vi "PH_SHS_Analysis_Statistician.panel.vi"(0 "object ref":refnum<vi>, 5 "error in (no error)":errorcluster) -> (19 "error out":errorcluster)   [LabVIEW 2014, in "PH_SHS_Analysis_Statistician.lvlib"]
doc: "This is just an example for a GUI thread.\n\nLicense Agreement for this software:\n\nCopyright (C)\nGesellschaft für Schwerionenforschung, GSI\nPlanckstr. 1\n64291 Darmstadt\nGermany\n\nContact: D.Beck@gsi.de \n\nThis program is free software; you can redistribute it and/or modify it under the terms of the GNU General Public License as published by the Free Software Foundation; either version 2 of the license, or (at your option) any later version.\n\nThis program is distributed in the hope that it will be useful, but WITHOUT ANYW ARRANTY; without even the implied warranty of MERCHANTABILITY or FITNESS FOR A PARTICULAR PURPOSE. See the GNU General License for more details (http://www.gnu.org).\n\nGesellschaft für Schwerionenforschung, GSI\nPlanckstr. 1, 64291 Darmstadt, Germany\nFor all questions and ideas contact: M.Richter@gsi.de, H.Brand@gsi.de or D.Beck@gsi.de.\nLast update: 18-DEC-2002"
uses:
  PH_SHS_Analysis_Statistician.lvlib
  PH_SHS_Analysis/PH_SHS_Analysis.Zernike Coefficients.ctl
  PH_Basics/PH_Common/PH_Common.lvlib
  CS_Core/CSSystem/CSSystemLib/CSSystemLib.lvlib
  PH_SHS_Analysis/PH_SHS_Analysis.lvlib
  PH_Basics/PH_Class/PH_Class.lvlib
panel:
  in  "Sample Length":i32=1
  in  "Clear Data":bool
  out "Current PtV [Lambda]":dbl
  out "Current Zernike Coefficients":T1 {"2nd Spherical" scale=-2.0..2.0 scale format="%.2f"; "2nd Coma y" scale=-2.0..2.0 scale format="%.2f"; "2nd Coma x" scale=-2.0..2.0 scale format="%.2f"; "2nd Astig 45°" scale=-2.0..2.0 scale format="%.2f"; "2nd Astig 0°" scale=-2.0..2.0 scale format="%.2f"; "Trefoil 30°" scale=-2.0..2.0 scale format="%.2f"; "Trefoil 0°" scale=-2.0..2.0 scale format="%.2f"; "Spherical" scale=-2.0..2.0 scale format="%.2f"; "Coma y" scale=-2.0..2.0 scale format="%.2f"; "Coma x" scale=-2.0..2.0 scale format="%.2f"; "Astig 45°" scale=-2.0..2.0 scale format="%.2f"; "Astig 0°" scale=-2.0..2.0 scale format="%.2f"; "Defocus" scale=-2.0..2.0 scale format="%.2f"; "Tilt y" scale=-2.0..2.0 scale format="%.2f"; "Tilt x" scale=-2.0..2.0 scale format="%.2f"}
  in  "Stat or Trend":bool
  in  "Export Data":bool
  out "Result Graph":cluster{dbl[], dbl[]}[](graph)
  out "Std Dev Data 3":dbl caption="Unit" format="%#_4g"
  in  "Dummy Std Dev":string caption="Std Dev"
  in  "Dummy Mean":string caption="Mean"
  out "Mean Data 3":dbl caption="Unit" format="%#_4g"
  out "Std Dev Data 2":dbl caption="Unit" format="%#_4g"
  out "Mean Data 2":dbl caption="Unit" format="%#_4g"
  out "Std Dev Data 1":dbl caption="Unit" format="%#_4g"
  out "Mean Data 1":dbl caption="Unit" format="%#_4g"
  in  "Data 3":u16(ring) items=["nothing "]
  in  "Data 2":u16(ring) items=["nothing "]
  in  "Data 1":u16(ring) items=["nothing "]
  out "Status":u32(colorbox)
  in  "Operator":string
  in  "Delete":bool
  # "PCS"
  # "3.40"
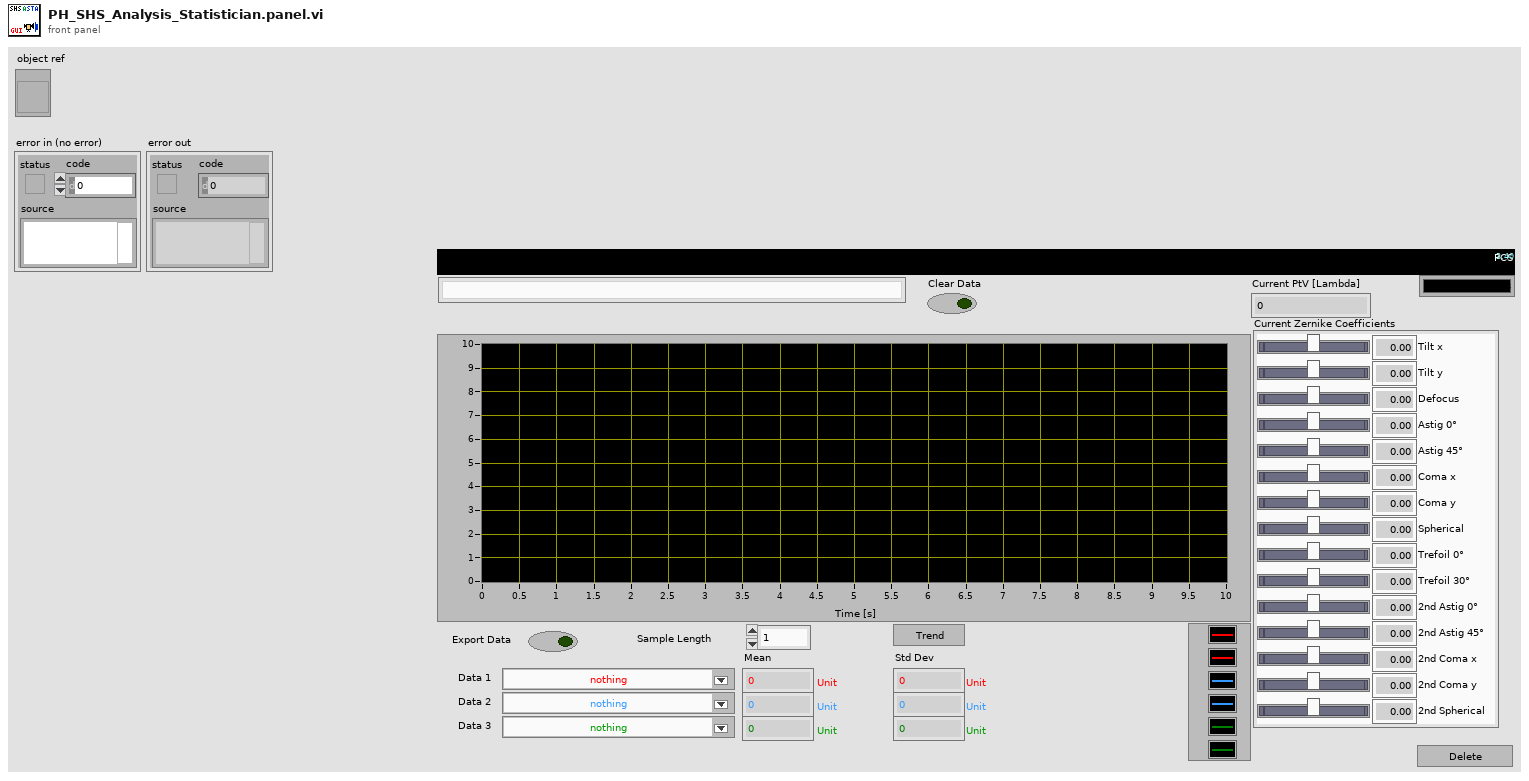
[diagram p1: front panel]
types:
  T1 = typedef "PH_SHS_Analysis.lvlib/PH_SHS_Analysis.Zernike Coefficients.ctl" = cluster{"Tilt x":dbl, "Tilt y":dbl, "Defocus":dbl, "Astig 0°":dbl, "Astig 45°":dbl, "Coma x":dbl, "Coma y":dbl, "Spherical":dbl, "Trefoil 0°":dbl, "Trefoil 30°":dbl, "2nd Astig 0°":dbl, "2nd Astig 45°":dbl, "2nd Coma x":dbl, "2nd Coma y":dbl, "2nd Spherical":dbl}
  T2 = enum8{"Enabled", "Disabled", "Disabled and Grayed Out"}
  T3 = typedef "PH_SHS_Analysis_Statistician.lvlib/PH_SHS_Analysis_Statistician.i attribute.ctl" = cluster{"GUI Refs ":cluster{"Status":refnum<vi>, "Result Graph":refnum<vi>, "Mean Data 1":refnum<vi>, "Std Dev Data 1":refnum<vi>, "Mean Data 2":refnum<vi>, "Std Dev Data 2":refnum<vi>, "Mean Data 3":refnum<vi>, "Std Dev Data 3":refnum<vi>, "Dummy Mean":refnum<vi>, "Dummy Std Dev":refnum<vi>, "Export Data":refnum<vi>, "Data 1":refnum<vi>, "Data 2":refnum<vi>, "Data 3":refnum<vi>, "Stat or Trend":refnum<vi>, "Delete":refnum<vi>, "Analyzer":refnum<vi>, "Current Zernike Coefficients":refnum<vi>, "PtV [Lambda]":refnum<vi>, "sample length":refnum<vi>}, "Analyzer":string, "Stat or Trend":bool, "Data 1":i16, "Data 2":i16, "Data 3":i16, "Data":T4[], "sample length":i32, "Datasets strored":i32, "Dataarray Size":i32}
  T4 = typedef "PH_SHS_Analysis.lvlib/PH_SHS_Analysis.Zernike Dataset.ctl" = cluster{"State":T5, "Time Stamp":timestamp, "PtV [lambda]":dbl, "Zernicke Coefficients":T1}
  T5 = typedef "PH_StatusHandler.lvlib/PH_StatusHandler.Status.ctl" = i16
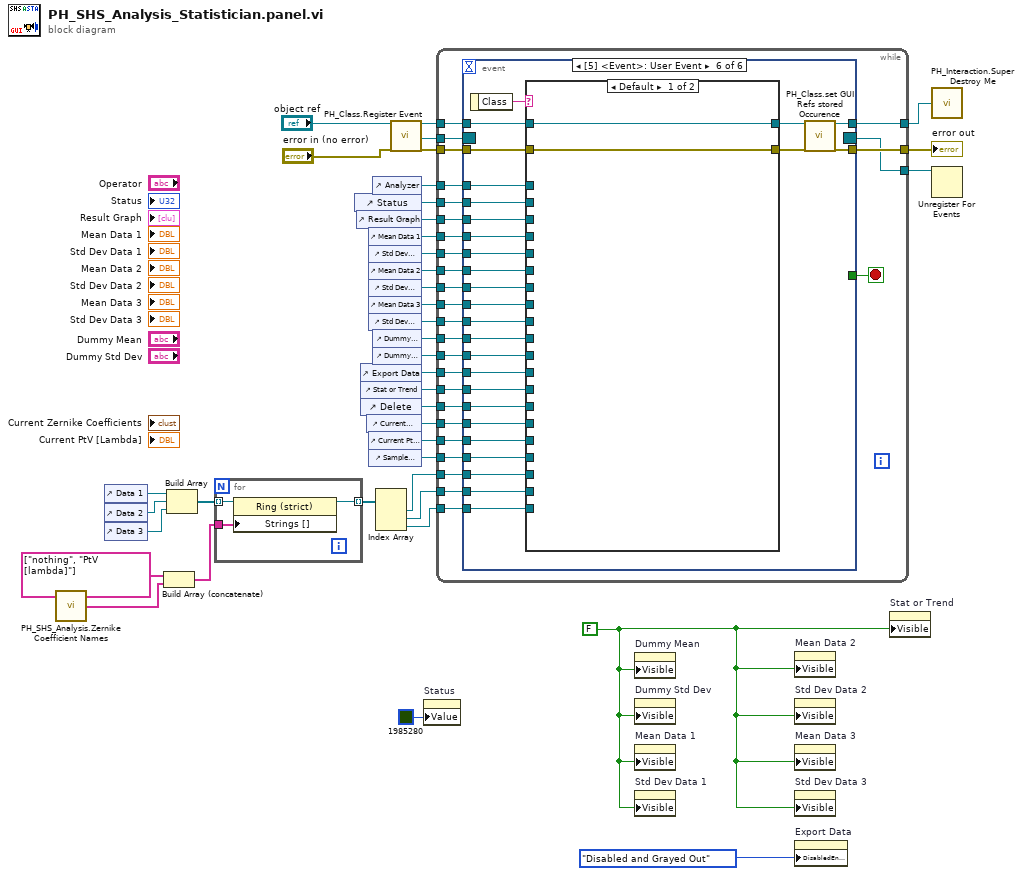
[diagram p0: block diagram]
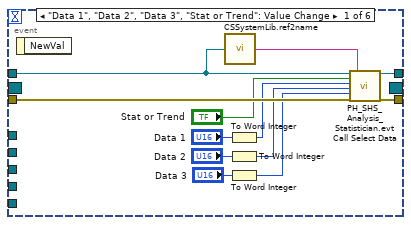
[diagram p2: hidden frame]
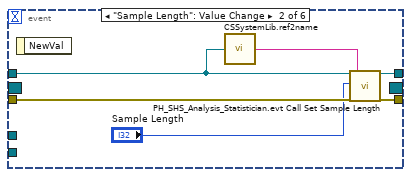
[diagram p3: hidden frame]
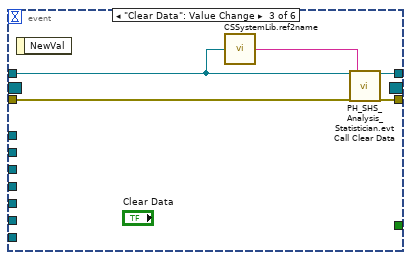
[diagram p4: hidden frame]
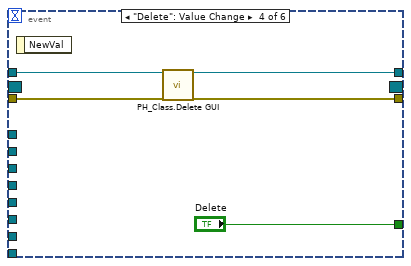
[diagram p5: hidden frame]
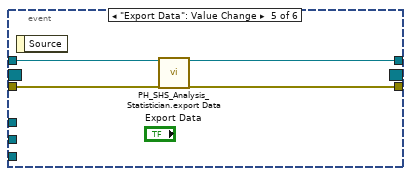
[diagram p6: hidden frame]
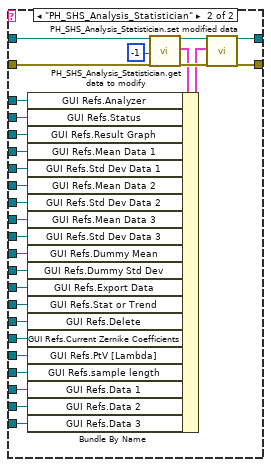
[diagram p7: hidden frame]
diagram:
  w36 = FALSE
  n1 = call "PH_SHS_Analysis.Zernike Coefficient Names.vi"() -> ("Zernickes"=w28:string[])
  n2 = control-ref of="Data 1"() -> (w39:refnum<vi>)
  n3 = control-ref of="Data 2"() -> (w31:refnum<vi>)
  n4 = control-ref of="Data 3"() -> (w30:refnum<vi>)
  n5 = Build Array (concatenate)(string[] ["nothing", "PtV [lambda]"], w28) -> (w27:string[])
  n6 = Build Array(w39, w31, w30) -> (w32:refnum<vi>[])
  n7 = for {
    tunnel: [w42] -> w33 mode=indexing
    tunnel: w32 -> [w41] mode=indexing
    tunnel: w27 -> [w40]
    n8 = property class="Ring (strict)"(reference=w41, "Strings []"=w40) -> (reference out=w42:refnum<vi>)  [unwired: 1 in, 1 out]
  }
  n9 = control-ref of="Status"() -> (w19:refnum<vi>)
  n10 = control-ref of="Result Graph"() -> (w18:refnum<vi>)
  n11 = control-ref of="Export Data"() -> (w9:refnum<vi>)
  n12 = control-ref of="Stat or Trend"() -> (w8:refnum<vi>)
  n13 = control-ref of="Delete"() -> (w7:refnum<vi>)
  n14 = control-ref of="Current Zernike Coefficients"() -> (w6:refnum<vi>)
  n15 = control-ref of="Mean Data 1"() -> (w17:refnum<vi>)
  n16 = control-ref of="Std Dev Data 1"() -> (w16:refnum<vi>)
  n17 = control-ref of="Mean Data 2"() -> (w15:refnum<vi>)
  n18 = control-ref of="Std Dev Data 2"() -> (w14:refnum<vi>)
  n19 = control-ref of="Mean Data 3"() -> (w13:refnum<vi>)
  n20 = control-ref of="Std Dev Data 3"() -> (w12:refnum<vi>)
  n21 = control-ref of="Current PtV [Lambda]"() -> (w5:refnum<vi>)
  n22 = control-ref of="Sample Length"() -> (w4:refnum<vi>)
  n23 = control-ref of="Analyzer"() -> (w20:refnum<vi>)
  n24 = control-ref of="Dummy Mean"() -> (w11:refnum<vi>)
  n25 = control-ref of="Dummy Std Dev"() -> (w10:refnum<vi>)
  n26 = Index Array(array=w33) -> (element #1=w3:refnum<vi>, element #2=w2:refnum<vi>, element #3=w1:refnum<vi>)  [unwired: 3 in]
  n27 = call "PH_Class.Register Event.vi"("i ref in"="object ref", "error in (no error)"="error in (no error)") -> ("i ref out"=w26:refnum<vi>, "Event Registration Refnum"=w24:refnum<event-registration>, "error out"=w25:errorcluster)  [unwired: 15 in]
  n28 = property on="Status" class="ColBox"("Value"=u32 1985280 ("Status")) -> ()  [unwired: 2 in, 2 out]
  n29 = while {
    tunnel: w26 -> [w68]
    tunnel: [w67] -> w38
    tunnel: [w66] -> w37
    tunnel: w25 -> [w65]
    tunnel: w24 -> [w64]
    tunnel: [w63] -> w23
    tunnel: w20 -> [w62]
    tunnel: w19 -> [w61]
    tunnel: w18 -> [w60]
    tunnel: w17 -> [w59]
    tunnel: w16 -> [w58]
    tunnel: w15 -> [w57]
    tunnel: w14 -> [w56]
    tunnel: w13 -> [w55]
    tunnel: w12 -> [w54]
    tunnel: w11 -> [w53]
    tunnel: w10 -> [w52]
    tunnel: w9 -> [w51]
    tunnel: w8 -> [w50]
    tunnel: w7 -> [w49]
    tunnel: w6 -> [w48]
    tunnel: w5 -> [w47]
    tunnel: w4 -> [w46]
    tunnel: w3 -> [w45]
    tunnel: w2 -> [w44]
    tunnel: w1 -> [w43]
    stop <- w69 stop-if-true
    n30 = event shown="[5] <Event>: User Event" {
      selector: w64 -> [_ _ _ _ _ _]
      dyn-events: [_ _ _ _ _ _] -> w63
      timeout: _ -> [_ _ _ _ _ _]
      tunnel: [_ _ _ "Delete" _ _] -> w69
      tunnel: w68 -> [w77 w83 w88 w96 w100 w126]
      tunnel: [w79 w85 w90 w95 w98 w128] -> w67
      tunnel: [w80 w86 w91 w93 w99 w127] -> w66
      tunnel: w65 -> [w81 w87 w92 w94 w101 w124]
      tunnel: w62 -> [_ _ _ _ _ w122]
      tunnel: w61 -> [_ _ _ _ _ w121]
      tunnel: w60 -> [_ _ _ _ _ w120]
      tunnel: w59 -> [_ _ _ _ _ w119]
      tunnel: w58 -> [_ _ _ _ _ w118]
      tunnel: w57 -> [_ _ _ _ _ w117]
      tunnel: w56 -> [_ _ _ _ _ w116]
      tunnel: w55 -> [_ _ _ _ _ w115]
      tunnel: w54 -> [_ _ _ _ _ w114]
      tunnel: w53 -> [_ _ _ _ _ w113]
      tunnel: w52 -> [_ _ _ _ _ w112]
      tunnel: w51 -> [_ _ _ _ _ w111]
      tunnel: w50 -> [_ _ _ _ _ w110]
      tunnel: w49 -> [_ _ _ _ _ w109]
      tunnel: w48 -> [_ _ _ _ _ w108]
      tunnel: w47 -> [_ _ _ _ _ w107]
      tunnel: w46 -> [_ _ _ _ _ w106]
      tunnel: w45 -> [_ _ _ _ _ w105]
      tunnel: w44 -> [_ _ _ _ _ w104]
      tunnel: w43 -> [_ _ _ _ _ w103]
      event "Data 1", "Data 2", "Data 3", "Stat or Trend": Value Change {
        n31 = event-data() -> ()  [unwired: 1 in, 1 out]
        n32 = call "CSSystemLib.ref2name.vi"("obj refnum"=w77) -> ("name"=w78:string)
        n33 = To Word Integer(number="Data 1") -> (16bit integer=w72:i16)
        n34 = To Word Integer(number="Data 2") -> (16bit integer=w71:i16)
        n35 = To Word Integer(number="Data 3") -> (16bit integer=w70:i16)
        n36 = call "PH_SHS_Analysis_Statistician.evt Call Select Data.vi"("i ref in"=w77, "Stat or Trend"="Stat or Trend", "Data 1"=w72, "Data 2"=w71, "Data 3"=w70, "error in (no error)"=w81, "Instance"=w78) -> ("i ref out"=w79:refnum<vi>, "error out"=w80:errorcluster)  [unwired: 11 in]
      }
      event "Sample Length": Value Change {
        n37 = event-data() -> ()  [unwired: 1 in, 1 out]
        n38 = call "CSSystemLib.ref2name.vi"("obj refnum"=w83) -> ("name"=w84:string)
        n39 = call "PH_SHS_Analysis_Statistician.evt Call Set Sample Length.vi"("i ref in"=w83, "Sample Length"="Sample Length", "error in (no error)"=w87, "Instance"=w84) -> ("i ref out"=w85:refnum<vi>, "error out"=w86:errorcluster)  [unwired: 14 in]
      }
      event "Clear Data": Value Change {
        n40 = event-data() -> ()  [unwired: 1 in, 1 out]
        n41 = call "CSSystemLib.ref2name.vi"("obj refnum"=w88) -> ("name"=w89:string)
        n42 = call "PH_SHS_Analysis_Statistician.evt Call Clear Data.vi"("i ref in"=w88, "error in (no error)"=w92, "Instance"=w89) -> ("i ref out"=w90:refnum<vi>, "error out"=w91:errorcluster)  [unwired: 15 in]
      }
      event "Delete": Value Change {
        n43 = event-data() -> ()  [unwired: 1 in, 1 out]
        n44 = call "PH_Class.Delete GUI.vi"("VI in"=w96, "error in (no error)"=w94) -> ("VI out"=w95:refnum<vi>, "error out"=w93:errorcluster)  [unwired: 16 in]
      }
      event "Export Data": Value Change {
        n45 = event-data() -> ()  [unwired: 1 in, 1 out]
        n46 = call "PH_SHS_Analysis_Statistician.export Data.vi"("i ref in"=w100, "error in (no error)"=w101) -> ("i ref out"=w98:refnum<vi>, "error out"=w99:errorcluster)  [unwired: 16 in]
      }
      event User Event {
        n47 = event-data() -> ("Class"=w102:string)  [unwired: 1 in]
        n48 = case shown="Default" w102 {
          tunnel: w126 -> [w130 w154]
          tunnel: [w130 w153] -> w125
          tunnel: w124 -> [w129 w152]
          tunnel: [w129 w151] -> w123
          tunnel: w122 -> [_ w150]
          tunnel: w121 -> [_ w149]
          tunnel: w120 -> [_ w148]
          tunnel: w119 -> [_ w147]
          tunnel: w118 -> [_ w146]
          tunnel: w117 -> [_ w145]
          tunnel: w116 -> [_ w144]
          tunnel: w115 -> [_ w143]
          tunnel: w114 -> [_ w142]
          tunnel: w113 -> [_ w141]
          tunnel: w112 -> [_ w140]
          tunnel: w111 -> [_ w139]
          tunnel: w110 -> [_ w138]
          tunnel: w109 -> [_ w137]
          tunnel: w108 -> [_ w136]
          tunnel: w107 -> [_ w135]
          tunnel: w106 -> [_ w134]
          tunnel: w105 -> [_ w133]
          tunnel: w104 -> [_ w132]
          tunnel: w103 -> [_ w131]
          frame Default {
          }
          frame "PH_SHS_Analysis_Statistician" {
            n49 = call "PH_SHS_Analysis_Statistician.get data to modify.vi"("i ref in"=w154, "ms timeout (10000)"=-1, "error in (no error)"=w152) -> ("i ref out"=w158:refnum<vi>, "i attribute"=w155:T3, "error out"=w159:errorcluster)  [unwired: 13 in, 1 out]
            n50 = Bundle By Name(cluster=w155, "GUI Refs.Analyzer"=w150, "GUI Refs.Status"=w149, "GUI Refs.Result Graph"=w148, "GUI Refs.Mean Data 1"=w147, "GUI Refs.Std Dev Data 1"=w146, "GUI Refs.Mean Data 2"=w145, "GUI Refs.Std Dev Data 2"=w144, "GUI Refs.Mean Data 3"=w143, "GUI Refs.Std Dev Data 3"=w142, "GUI Refs.Dummy Mean"=w141, "GUI Refs.Dummy Std Dev"=w140, "GUI Refs.Export Data"=w139, "GUI Refs.Stat or Trend"=w138, "GUI Refs.Delete"=w137, "GUI Refs.Current Zernike Coefficients"=w136, "GUI Refs.PtV [Lambda]"=w135, "GUI Refs.sample length"=w134, "GUI Refs.Data 1"=w133, "GUI Refs.Data 2"=w132, "GUI Refs.Data 3"=w131) -> (w156:T3)
            n51 = call "PH_SHS_Analysis_Statistician.set modified data.vi"("i ref in"=w158, "i attribute"=w156, "error in (no error)"=w159) -> ("i ref out"=w153:refnum<vi>, "error out"=w151:errorcluster)  [unwired: 15 in]
          }
        }
        n52 = call "PH_Class.set GUI Refs stored Occurence.vi"("i ref in"=w125, "error in (no error)"=w123) -> ("i ref out"=w128:refnum<vi>, "error out"=w127:errorcluster)  [unwired: 16 in]
      }
    }
  }
  "error out" <- w37
  n53 = property on="Dummy Mean" class="Str"("Visible"=w36) -> ()  [unwired: 2 in, 2 out]
  n54 = property on="Dummy Std Dev" class="Str"("Visible"=w36) -> ()  [unwired: 2 in, 2 out]
  n55 = property on="Mean Data 1" class="DigNum (strict)"("Visible"=w36) -> ()  [unwired: 2 in, 2 out]
  n56 = property on="Std Dev Data 1" class="DigNum (strict)"("Visible"=w36) -> ()  [unwired: 2 in, 2 out]
  n57 = property on="Mean Data 2" class="DigNum (strict)"("Visible"=w36) -> ()  [unwired: 2 in, 2 out]
  n58 = property on="Std Dev Data 2" class="DigNum (strict)"("Visible"=w36) -> ()  [unwired: 2 in, 2 out]
  n59 = property on="Mean Data 3" class="DigNum (strict)"("Visible"=w36) -> ()  [unwired: 2 in, 2 out]
  n60 = property on="Std Dev Data 3" class="DigNum (strict)"("Visible"=w36) -> ()  [unwired: 2 in, 2 out]
  n61 = property on="Export Data" class="Bool"("DisabledEnum"=T2."Disabled and Grayed Out" ("Disabled")) -> ()  [unwired: 2 in, 2 out]
  n62 = property on="Stat or Trend" class="Bool (strict)"("Visible"=w36) -> ()  [unwired: 2 in, 2 out]
  n63 = call "PH_Interaction.Super Destroy Me.vi"("i ref out"=w38) -> ()
  n64 = Unregister For Events(event registration refnum=w23) -> ()  [unwired: 1 in, 1 out]
